vi "LowPassAccelData.vi"(1 "alpha":dbl=0.5 format="%#_13g", 2 "Prev Gs":T1, 3 "Input Gs":T1) -> (0 "G-Filtered":T1)   [LabVIEW 2015]
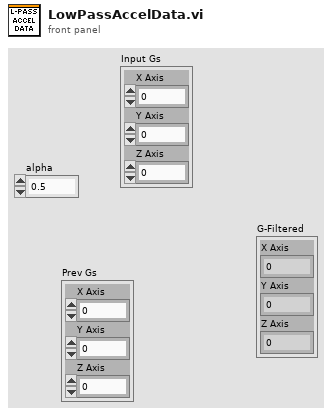
[diagram p1: front panel]
types:
  T1 = cluster{"X Axis":dbl, "Y Axis":dbl, "Z Axis":dbl}
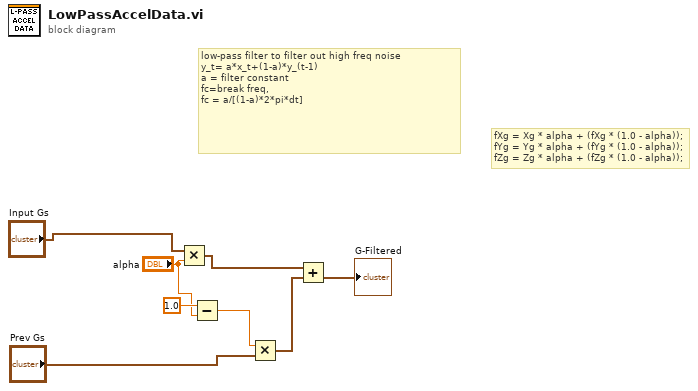
[diagram p0: block diagram]
diagram:
  # "fXg = Xg * alpha + (fXg * (1.0 - alpha));\nfYg = Yg * alpha + (fYg * (1.0 - alpha));\nfZg = Zg * alpha + (fZg * (1.0 - alpha));"
  # "low-pass filter to filter out high freq noise\ny_t= a*x_t+(1-a)*y_(t-1)\na = filter constant\nfc=break freq,\nfc = a/[(1-a)*2*pi*dt]"
  n1 = Multiply(x="Input Gs", y="alpha") -> (x*y=w3:T1)
  n2 = Subtract(x=1.0, y="alpha") -> (x-y=w6:dbl)
  n3 = Multiply(x=w6, y="Prev Gs") -> (x*y=w4:T1)
  n4 = Add(x=w3, y=w4) -> (x+y=→"G-Filtered":T1)
